vi "2.1.带Reset的计数器.vi"() -> ()   [LabVIEW 2019]
uses:
  <vilib>/rvi/Emulation/niFpgaGetClockAttributes.vi
  <vilib>/rvi/Emulation/niFpgaSctlEmulationGetInTimedLoop.vi
  <vilib>/rvi/Emulation/niFpgaEmulationReportErrorSimple.vi
  <vilib>/rvi/eio/common/nirviEmuTemplateMethod_errors.vi
  <vilib>/rvi/Emulation/niFpgaCriticalErrorInLSC.vi
  <vilib>/eio/EIONode/EIONode.xnode
panel:
  out "数值":u32
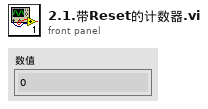
[diagram p1: front panel]
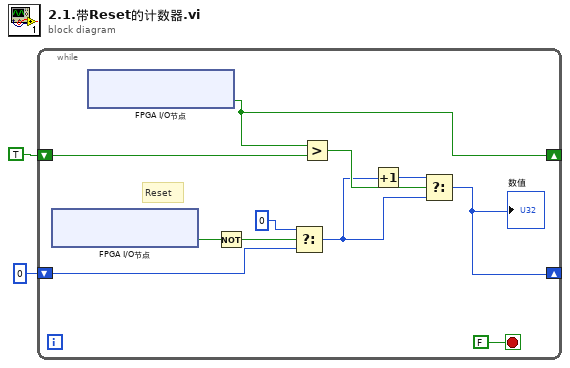
[diagram p0: block diagram]
diagram:
  n1 = while {
    shift-right: [w5] -> _
    shift-left: u32 0 -> [w12]
    shift-right: [w10] -> _
    shift-left: TRUE -> [w11]
    stop <- FALSE stop-if-true
    # "Reset"
    n2 = xnode "FPGA I/O节点"() -> ("ConnectorA/DIO1"=w4:bool)  [unwired: 1 in, 1 out]
    n3 = xnode "FPGA I/O节点"() -> ("ConnectorA/DIO0"=w10:bool)  [unwired: 1 in, 1 out]
    n4 = Not(x=w4) -> (.not. x?=w3:bool)
    n5 = Select(t=u32 0, s=w3, f=w12) -> (s? t:f=w7:u32)
    n6 = Greater?(x=w10, y=w11) -> (0:w9:bool)
    n7 = Increment(x=w7) -> (x+1=w8:u32)
    n8 = Select(t=w8, s=w9, f=w7) -> (s? t:f=w5:u32)
    "数值" <- w5
  }
